vi "Set Phosphor Event.vi"(11 "driverEvent":u32) -> (2 "function return":u32, 3 "driverEvent out":u32)   [LabVIEW 2018, in "AndorSDK.lvlib"]
doc: "EXPNETTYPE unsigned int WINAPI SetPhosphorEvent(HANDLE driverEvent);"
uses:
  AndorSDK.lvlib
  ATMCD32D.dll
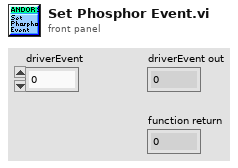
[diagram p1: front panel]
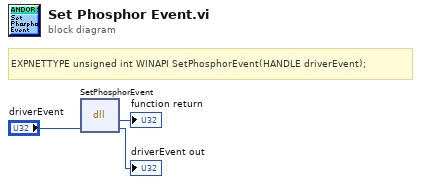
[diagram p0: block diagram]
diagram:
  # "EXPNETTYPE unsigned int WINAPI SetPhosphorEvent(HANDLE driverEvent);"
  n1 = dll-call lib="PTH2babs E\nPersönliches02 - Arbeit03-HiwijobsLabviewCodelibANDOR\tAndor SDK\nATMCD32D.*" fn="SetPhosphorEvent"("driverEvent"="driverEvent") -> (→"function return":u32, "driverEvent"=→"driverEvent out":u32)  [unwired: 3 in, 2 out]
